vi "Load Shared Variable File.vi"(8 "error in":errorcluster, 11 "Device Ref in":T1 format="%.0x") -> (0 "error out":errorcluster, 3 "Device Ref out":T1 format="%.0x")   [LabVIEW 2017, in "Shared Variables CD 2.0 Configuration.lvlib"]
uses:
  Shared Variables CD 2.0 Configuration.lvlib
  <vilib>/NI Veristand/Custom Device API/Custom Device Item Ref.ctl
  <vilib>/Utility/VariantDataType/Type.ctl
  <vilib>/NI Veristand/Custom Device API/Custom Device Channel.ctl
  <vilib>/NI Veristand/Custom Device API/Custom Device Channel Type.ctl
  <userlib>/_OpenG.lib/file/file.llb/Valid Path - Traditional__ogtk.vi
  Shared/SV Global.vi
  Shared/Shared Variables CD 2.0 GUID Lookup.vi
  <vilib>/Utility/VariantDataType/VariantType.lvlib
  <vilib>/NI Veristand/Custom Device API/Custom Device API.lvlib
panel:
  in  "Cancel Button":bool
  in  "OK Button":bool
  in  "Shared Variable File Path":path
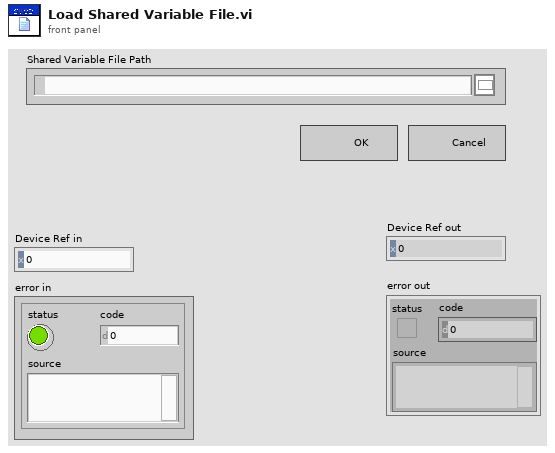
[diagram p1: front panel]
types:
  T1 = typedef "Custom Device API.lvlib/Custom Device Item Ref.ctl" = u64
  T2 = typedef "Custom Device API.lvlib/Custom Device Channel.ctl" = cluster{"Type":T3, "Units":string, "Default Value":dbl, "Faultable":bool, "Scalable":bool}
  T3 = typedef "Custom Device API.lvlib/Custom Device Channel Type.ctl" = enum16{"Input", "Output"}
  T4 = typedef "VariantType.lvlib/Type.ctl" = enum8{"Invalid Type", "Void", "I8", "I16", "I32", "I64", "U8", "U16", "U32", "U64", "Single Float", "Double Float", "Extended Float", "Single Complex", "Double Complex", "Extended Complex", "Enum U8", "Enum U16", "Enum U32", "Enum U64", "Single Float With Unit", "Double Float With Unit", "Extended Float With Unit", "Single Complex with Unit", "Double Complex with Unit", "Extended Complex with Unit", "Boolean", "String", "Path", "Picture", "Tag", "Array", "Cluster", "Variant", "LV Variant", "Waveform", "Timestamp", "Digital Waveform", "Digital Data", "ExpressData", "Refnum", "External Data", "VI", "Poly VI", "LabVIEW Class Instance", "Fixed Point"}
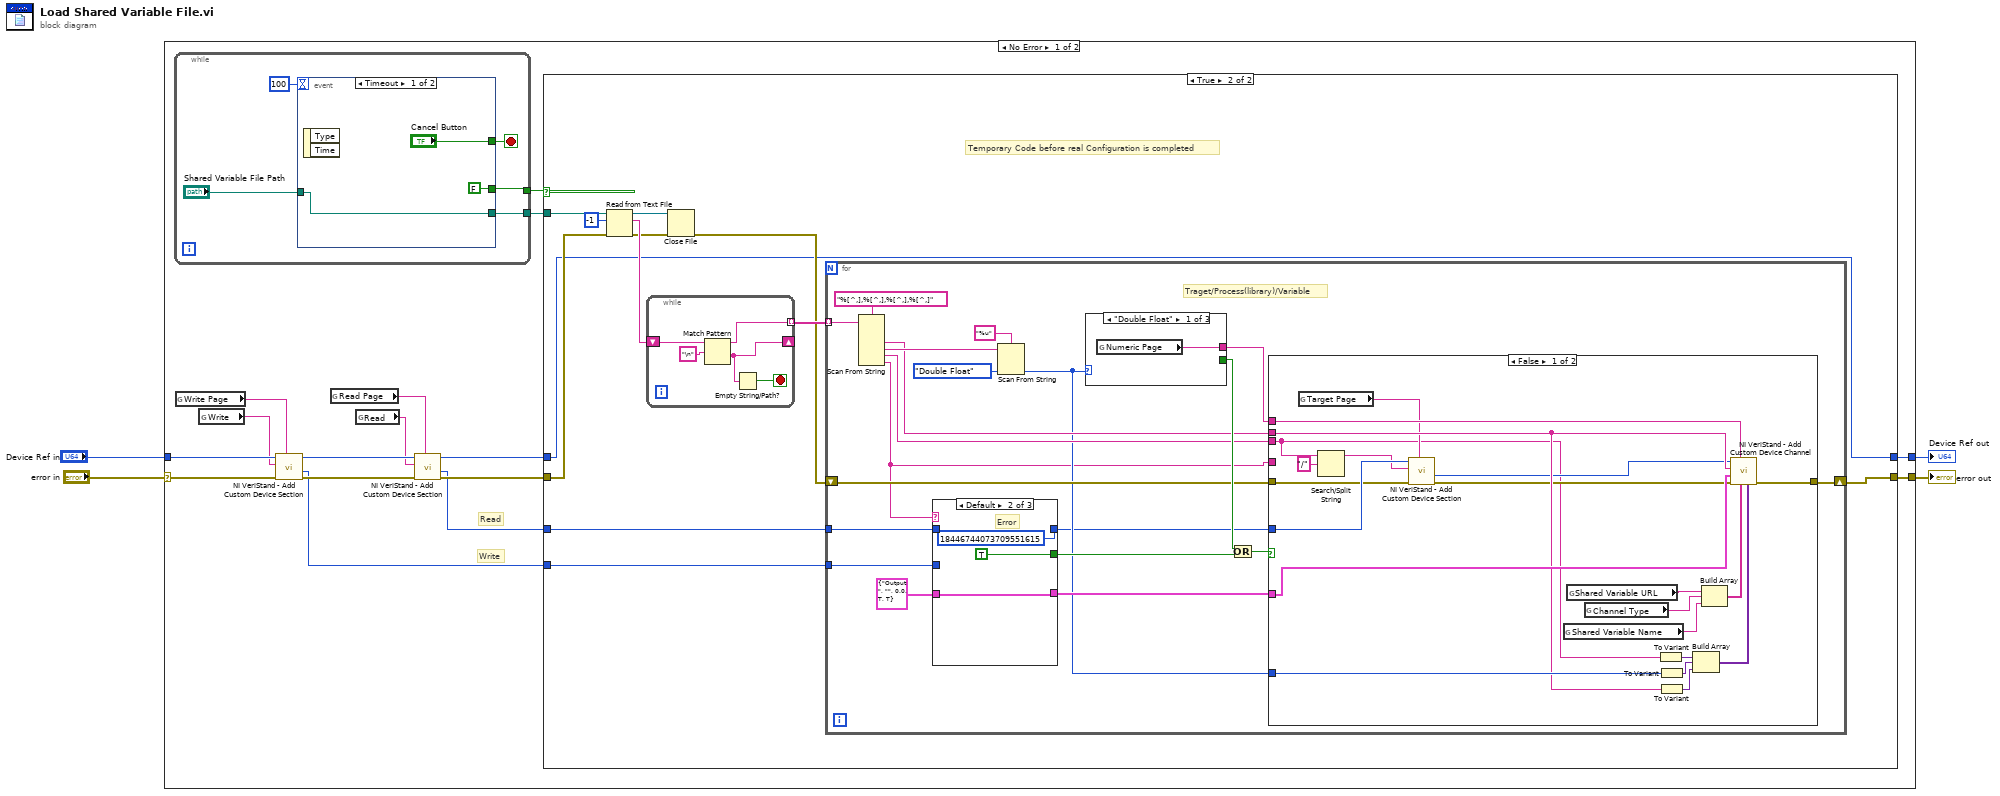
[diagram p0: block diagram]
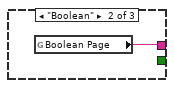
[diagram p3: hidden frame]
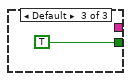
[diagram p4: hidden frame]
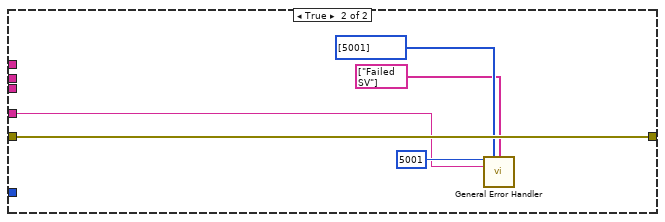
[diagram p5: hidden frame]
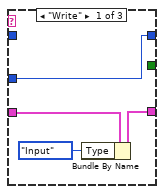
[diagram p6: hidden frame]
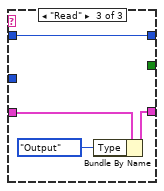
[diagram p7: hidden frame]
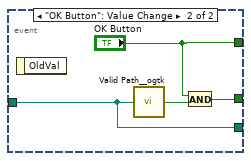
[diagram p8: hidden frame]
diagram:
  n1 = case shown="No Error" "error in" {
    selector: "error in" -> [w12 w113]
    tunnel: "Device Ref in" -> [w15 w112]
    tunnel: [w18 w113] -> w3
    tunnel: [w17 w112] -> w1
    frame No Error {
      # "Write"
      # "Read"
      n2 = while {
        tunnel: [w101] -> w19
        tunnel: [w100] -> w20
        stop <- w102 stop-if-true
        n3 = event shown="[0] Timeout" {
          selector: _ -> [_ _]
          dyn-events: _ -> [_ _]
          timeout: 100 -> [_ _]
          tunnel: "Shared Variable File Path" -> [w105 w108]
          tunnel: [FALSE w110] -> w100
          tunnel: ["Cancel Button" "OK Button"] -> w102
          tunnel: [w105 w108] -> w101
          event Timeout {
            n4 = event-data() -> ()  [unwired: 1 in, 2 out]
          }
          event "OK Button": Value Change {
            n5 = event-data() -> ()  [unwired: 1 in, 1 out]
            n6 = call-poly <userlib>:"Valid Path__ogtk.vi"("path"=w108) -> ("valid"=w111:bool)
            n7 = And(x="OK Button", y=w111) -> (x .and. y?=w110:bool)
          }
        }
      }
      n8 = global read "Shared Variables CD 2.0 GUID Lookup.vi" "Write Page"() -> (w6:string)
      n9 = global read "SV Global.vi" "Write"() -> (w7:string)
      n10 = call <vilib>:"NI VeriStand - Add Custom Device Section.vi"("GUID (Default Section)"=w6, "error in (no error)"=w12, "Section Name"=w7, "Parent Ref in"=w15) -> ("error out"=w13:errorcluster, "Section Ptr"=w8:T1, "Parent Ref out"=w16:T1)  [unwired: 4 in, 1 out]
      n11 = global read "Shared Variables CD 2.0 GUID Lookup.vi" "Read Page"() -> (w5:string)
      n12 = global read "SV Global.vi" "Read"() -> (w10:string)
      n13 = call <vilib>:"NI VeriStand - Add Custom Device Section.vi"("GUID (Default Section)"=w5, "error in (no error)"=w13, "Section Name"=w10, "Parent Ref in"=w16) -> ("error out"=w11:errorcluster, "Section Ptr"=w9:T1, "Parent Ref out"=w14:T1)  [unwired: 4 in, 1 out]
      n14 = case shown="True" w20 {
        tunnel: w19 -> [_ w34]
        tunnel: w11 -> [w22 w32]
        tunnel: [w22 w26] -> w18
        tunnel: w14 -> [w21 w23]
        tunnel: [w21 w23] -> w17
        tunnel: w9 -> [_ w25]
        tunnel: w8 -> [_ w24]
        frame False {
        }
        frame True {
          # "Temporary Code before real Configuration is completed"
          n15 = Read from Text File(file (use dialog)=w34, count=-1, error in=w32) -> (refnum out=w29:refnum<file>, text=w31:string, error out=w30:errorcluster)  [unwired: 1 in, 1 out]
          n16 = while {
            shift-right: [w96] -> _
            shift-left: w31 -> [w99]
            tunnel: [w97] -> w28 mode=indexing
            stop <- w95 stop-if-true
            n17 = Match Pattern(string=w99, regular expression="\n") -> (before substring=w97:string, after substring=w96:string)  [unwired: 1 in, 2 out]
            n18 = Empty String/Path?(string/path=w96) -> (empty?=w95:bool)
          }
          n19 = Close File(refnum=w29, error in=w30) -> (error out=w27:errorcluster)  [unwired: 1 out]
          n20 = for {
            tunnel: w28 -> [w54] mode=indexing
            shift-right: [w40] -> w26
            shift-left: w27 -> [w43]
            tunnel: w25 -> [w38]
            tunnel: w24 -> [w39]
            # "Traget/Process(library)/Variable"
            n21 = Scan From String(format string="%[^,],%[^,],%[^,],%[^,]", input string=w54) -> (output 1=w46:string, output 2=w50:string, output 3=w42:string, output 4=w35:string)  [unwired: 6 in, 3 out]
            n22 = case shown="Default" w35 {
              tunnel: [_ TRUE _] -> w48
              tunnel: T2 {"Type"=enum."Output", "Units"="", "Default Value"=0.0, "Faultable"=TRUE, "Scalable"=TRUE} ("Channel") -> [w87 w89 w94]
              tunnel: [w85 w89 w92] -> w44
              tunnel: w39 -> [w84 _ _]
              tunnel: w38 -> [_ _ w91]
              tunnel: [w84 T1 18446744073709551615 ("Section Ptr") w91] -> w36
              frame "Write" {
                n23 = Bundle By Name(cluster=w87, "Type"=Custom_Device_Channel_Type."Input") -> (w85:T2)
              }
              frame Default {
                # "Error"
              }
              frame "Read" {
                n24 = Bundle By Name(cluster=w94, "Type"=Custom_Device_Channel_Type."Output") -> (w92:T2)
              }
            }
            n25 = Scan From String(format string="%u", input string=w50, default 1=Type."Double Float" ("Type Enum")) -> (output 1=w41:T4)  [unwired: 2 in, 3 out]
            n26 = case shown="\"Double Float\"" w41 {
              tunnel: [_ _ TRUE] -> w49
              tunnel: [w55 w56 _] -> w47
              frame "Double Float" {
                n27 = global read "Shared Variables CD 2.0 GUID Lookup.vi" "Numeric Page"() -> (w55:string)
              }
              frame "Boolean" {
                n28 = global read "Shared Variables CD 2.0 GUID Lookup.vi" "Boolean Page"() -> (w56:string)
              }
              frame Default {
              }
            }
            n29 = Or(x=w49, y=w48) -> (x .or. y?=w37:bool)
            n30 = case shown="False" w37 {
              tunnel: w47 -> [w78 _]
              tunnel: w46 -> [w70 _]
              tunnel: w44 -> [w77 _]
              tunnel: w43 -> [w66 w83]
              tunnel: w42 -> [w63 _]
              tunnel: w41 -> [w71 _]
              tunnel: [w69 w83] -> w40
              tunnel: w36 -> [w68 _]
              tunnel: w35 -> [_ w79]
              frame False {
                n31 = global read "Shared Variables CD 2.0 GUID Lookup.vi" "Target Page"() -> (w64:string)
                n32 = Search/Split String(string=w63, search string/char (-)="/") -> (substring before match=w62:string)  [unwired: 1 in, 2 out]
                n33 = call <vilib>:"NI VeriStand - Add Custom Device Section.vi"("GUID (Default Section)"=w64, "error in (no error)"=w66, "Section Name"=w62, "Parent Ref in"=w68) -> ("error out"=w65:errorcluster, "Section Ptr"=w67:T1)  [unwired: 4 in, 2 out]
                n34 = global read "SV Global.vi" "Shared Variable Name"() -> (w59:string)
                n35 = global read "SV Global.vi" "Shared Variable URL"() -> (w60:string)
                n36 = global read "SV Global.vi" "Channel Type"() -> (w58:string)
                n37 = To Variant(anything=w63) -> (Variant=w75:variant)
                n38 = To Variant(anything=w71) -> (Variant=w74:variant)
                n39 = To Variant(anything=w70) -> (Variant=w72:variant)
                n40 = Build Array(w75, w74, w72) -> (w73:variant[])
                n41 = Build Array(w60, w58, w59) -> (w76:string[])
                n42 = call <vilib>:"NI VeriStand - Add Custom Device Channel.vi"("Property Values"=w73, "Property names"=w76, "GUID (Default Channel)"=w78, "error in (no error)"=w65, "Channel"=w77, "Channel Name"=w70, "Parent Ref in"=w67) -> ("error out"=w69:errorcluster)  [unwired: 1 in, 3 out]
              }
              frame True {
                n43 = call <vilib>:"General Error Handler.vi"("[error code] (0)"=5001, "[user-defined codes]"=i32[] [5001], "[user-defined descriptions]"=string[] ["Failed SV"], "[error source] (\" \")"=w79) -> ()  [unwired: 7 in, 5 out]
              }
            }
          }
        }
      }
    }
    frame Error {
    }
  }
  "error out" <- w3
  "Device Ref out" <- w1
